vi "getTestsFromTestCase.vi"(8 "error in":errorcluster, 10 "TestCase Name":string) -> (0 "error out":errorcluster, 1 "test paths":path[](array[path]), 2 "tests":string[](array[string]))   [LabVIEW 2013, in "TestLoader.lvclass"]
uses:
  TestLoader.lvclass
panel:
  # "JKI VI Tester for LabVIEW\nhttp://jkisoft.com/vi-tester\nCopyright (C) 2007-2009, JKI <info@jkisoft.com>\nALL RIGHTS RESERVED"
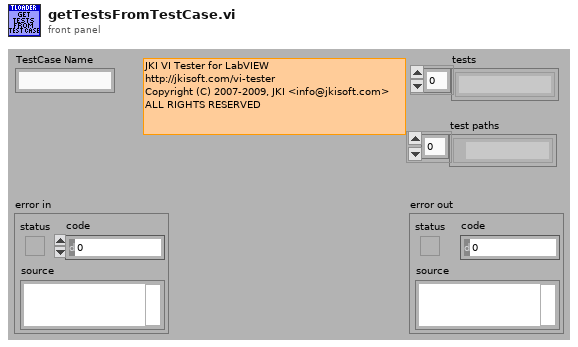
[diagram p1: front panel]
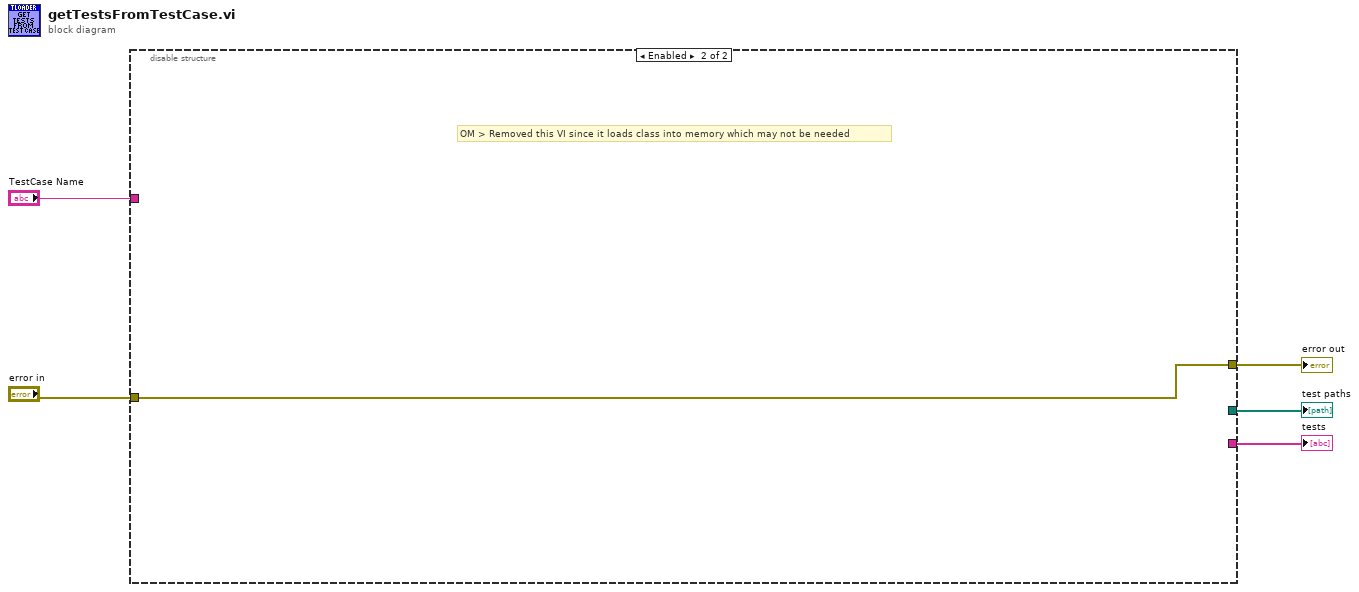
[diagram p0: block diagram]
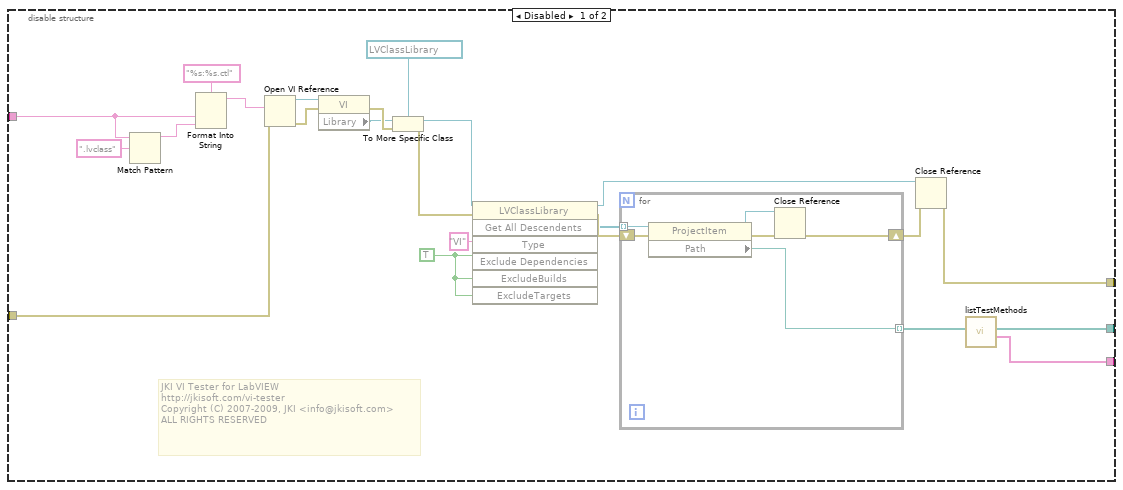
[diagram p2: hidden frame]
diagram:
  n1 = disable-structure shown="Enabled" {
    disable-tunnel: [w28 w35] -> w5
    disable-tunnel: "error in" -> [w14 w35]
    disable-tunnel: "TestCase Name" -> [w11 _]
    disable-tunnel: [w7 _] -> w2
    disable-tunnel: [w6 _] -> w1
    frame Disabled {
      w9 = TRUE ("ExcludeDependencies")
      # "JKI VI Tester for LabVIEW\nhttp://jkisoft.com/vi-tester\nCopyright (C) 2007-2009, JKI <info@jkisoft.com>\nALL RIGHTS RESERVED"
      n2 = Match Pattern(string=w11, regular expression=".lvclass") -> (before substring=w15:string)  [unwired: 1 in, 3 out]
      n3 = Format Into String(format string="%s:%s.ctl", w11, w15) -> (resulting string=w13:string)  [unwired: 2 in, 1 out]
      n4 = Open VI Reference(vi path=w13, error in (no error)=w14) -> (vi reference=w16:refnum<vi>, error out=w19:errorcluster)  [unwired: 4 in]
      n5 = property class="VI"(reference=w16, error in=w19) -> (error out=w20:errorcluster, "Library"=w17:refnum<vi>)  [unwired: 1 out]
      n6 = To More Specific Class(target class=refnum<vi> refnum ("Library"), reference=w17, error in=w20) -> (specific class reference=w21:refnum<vi>, error out=w25:errorcluster)
      n7 = invoke class="LVClassLibrary" method="Get All Descendents"(reference=w21, error in=w25, "Type"="VI", "Exclude Dependencies"=w9, "ExcludeBuilds"=w9, "ExcludeTargets"=w9) -> (reference out=w26:refnum<vi>, error out=w24:errorcluster, "All Descendents"=w23:refnum<vi>[])  [unwired: 1 in, 4 out]
      n8 = for {
        tunnel: w23 -> [w34] mode=indexing
        shift-right: [w30] -> w27
        shift-left: w24 -> [w33]
        tunnel: [w29] -> w8 mode=indexing
        n9 = property class="ProjectItem"(reference=w34, error in=w33) -> (reference out=w32:refnum<vi>, error out=w31:errorcluster, "Path"=w29:path)
        n10 = Close Reference(reference=w32, error in (no error)=w31) -> (error out=w30:errorcluster)
      }
      n11 = Close Reference(reference=w26, error in (no error)=w27) -> (error out=w28:errorcluster)
      n12 = call "listTestMethods.vi"("Methods"=w8) -> ("Test Method Names"=w6:string[], "Test Method Paths"=w7:path[])  [unwired: 9 in]
    }
    frame Enabled {
      # "OM > Removed this VI since it loads class into memory which may not be needed"
    }
  }
  "error out" <- w5
  "tests" <- w1
  "test paths" <- w2
